vi "BusB Raw Data.vi"(8 "error in (no error)":errorcluster, 10 "BusB Raw Data":u8[](array[numeric])) -> (0 "error out":errorcluster)   [LabVIEW 2016, in "Impedance Data Acquisition and Decoding.lvlib"]
doc: "_____\nCreated using Delacor QMH Event Scripter 5.0.0.112."
uses:
  Impedance Data Acquisition and Decoding.lvlib
  BusB Raw Data Argument--cluster.ctl
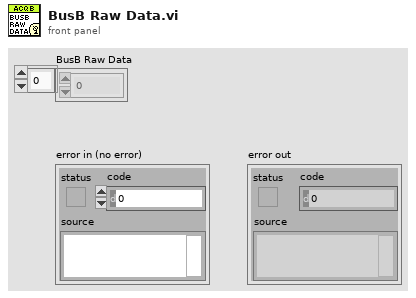
[diagram p1: front panel]
types:
  T1 = typedef "Impedance Data Acquisition and Decoding.lvlib/BusB Raw Data Argument--cluster.ctl" = cluster{"BusB Raw Data":u8[]}
  T2 = typedef "Impedance Data Acquisition and Decoding.lvlib/Broadcast Events--cluster.ctl" = cluster{"Module Did Init":refnum<user-event>, "Status Updated":refnum<user-event>, "Error Reported":refnum<user-event>, "Module Did Stop":refnum<user-event>, "Update Module Execution Status":refnum<user-event>, "Acquisition Stopped":refnum<user-event>, "BusB Raw Data":refnum<user-event>, "BusB Decoded Data Updated":refnum<user-event>, "Acquisition Started":refnum<user-event>, "Read Timeout Error Generation":refnum<user-event>}
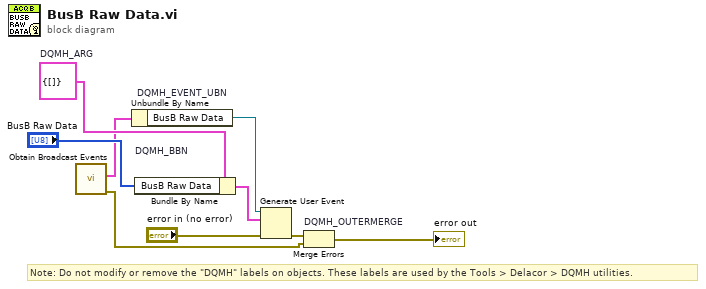
[diagram p0: block diagram]
diagram:
  w4 = T1 {"BusB Raw Data"=[]}  # DQMH_ARG
  # "Note: Do not modify or remove the \"DQMH\" labels on objects. These labels are used by the Tools > Delacor > DQMH utilities."
  n1 = call "Obtain Broadcast Events.vi"() -> ("error out"=w2:errorcluster, "FINS3-E BusB Data Acquisition and Decoding Broadcast Events"=w1:T2)  [unwired: 10 in]
  n2 = Unbundle By Name "DQMH_EVENT_UBN"(w1) -> ("BusB Raw Data"=w6:refnum<user-event>)
  n3 = Bundle By Name "DQMH_BBN"(cluster=w4, "BusB Raw Data"="BusB Raw Data") -> (w7:T1)
  n4 = Generate User Event(user event=w6, event data cluster=w7, error in="error in (no error)") -> (error out=w5:errorcluster)  [unwired: 1 in, 1 out]
  n5 = Merge Errors "DQMH_OUTERMERGE"(w5, w2) -> (→"error out":errorcluster)
